vi "Read Dashboard Values.vi"() -> ()   [LabVIEW 2020]
uses:
  <vilib>/Rock Robotics/Network Tables/NT Read Number.vi
  Framework/Robot Global Data.vi
panel:
  out "Auto Drive Time":dbl=3.0 format="%#_13g"
  out "Auto Right Speed":dbl=0.5 format="%#_13g"
  out "Auto Left Speed":dbl=0.5 format="%#_13g"
  out "Auto Shoot Time":dbl=1.0 format="%#_13g"
  out "Auto Shoot Set":dbl=-0.25 format="%#_13g"
  out "Shooter Duration (s)":dbl=3.0 format="%#_13g"
  out "Shooter Setpoint":dbl=0.8 format="%#_13g"
  out "Intake Duration (s)":dbl=3.0 format="%#_13g"
  out "Intake Setpoint":dbl=0.8 format="%#_13g"
  out "Pivot Right Setpoint":dbl=0.4 format="%#_13g"
  out "Pivot Left Setpoint":dbl=0.3 format="%#_13g"
  out "Control Panel Duration (s)":dbl=3.0 format="%#_13g"
  out "Control Panel Setpoint":dbl=0.8 format="%#_13g"
  out "CIimb Duration (s)":dbl=3.0 format="%#_13g"
  out "CIimb Setpoint":dbl=0.8 format="%#_13g"
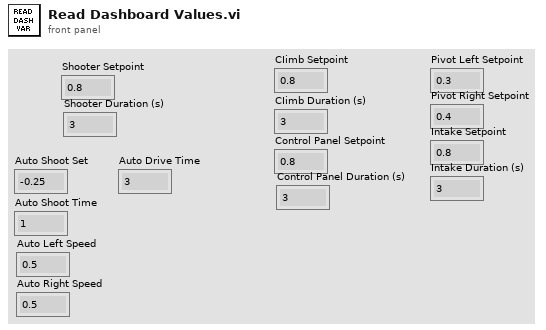
[diagram p1: front panel]
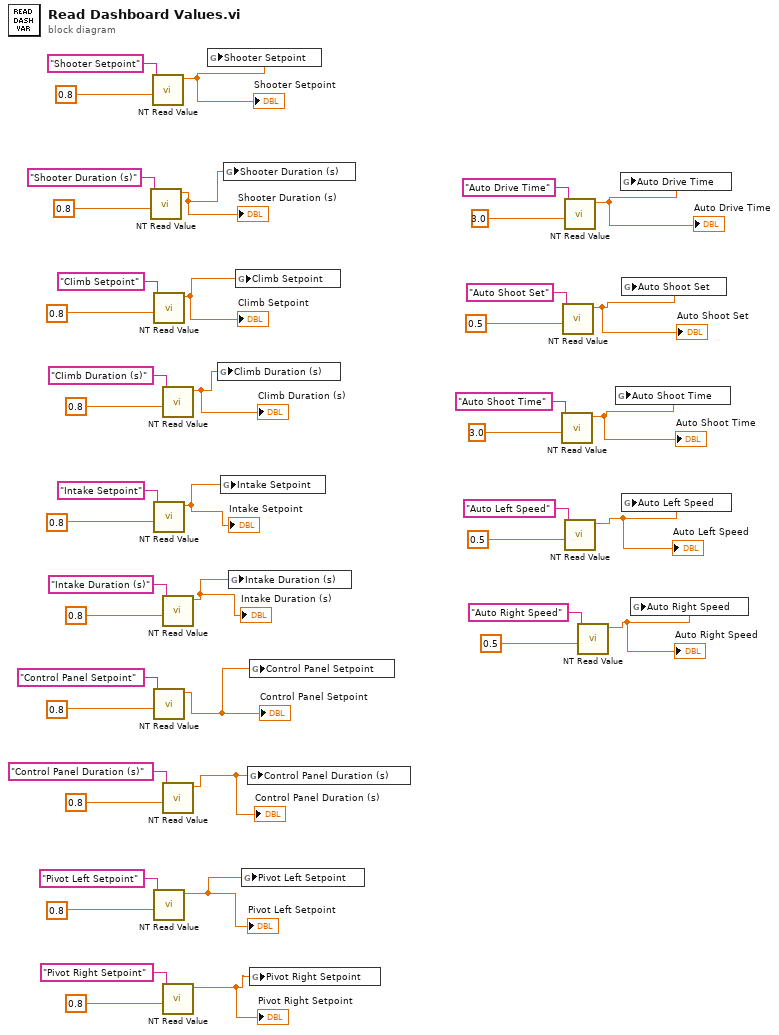
[diagram p0: block diagram]
diagram:
  n1 = call-poly <vilib>:"NT Read Value.vi"("Default Value"=0.8, "Name"="Shooter Duration (s)") -> ("Numeric"=w40:dbl)  [unwired: 8 in, 1 out]
  "Shooter Duration (s)" <- w40
  n2 = call-poly <vilib>:"NT Read Value.vi"("Default Value"=0.8, "Name"="Shooter Setpoint") -> ("Numeric"=w43:dbl)  [unwired: 8 in, 1 out]
  "Shooter Setpoint" <- w43
  n3 = call-poly <vilib>:"NT Read Value.vi"("Default Value"=0.8, "Name"="CIimb Setpoint") -> ("Numeric"=w35:dbl)  [unwired: 8 in, 1 out]
  "CIimb Setpoint" <- w35
  n4 = call-poly <vilib>:"NT Read Value.vi"("Default Value"=0.8, "Name"="Intake Setpoint") -> ("Numeric"=w21:dbl)  [unwired: 8 in, 1 out]
  "Intake Setpoint" <- w21
  n5 = call-poly <vilib>:"NT Read Value.vi"("Default Value"=0.8, "Name"="Control Panel Setpoint") -> ("Numeric"=w18:dbl)  [unwired: 8 in, 1 out]
  "Control Panel Setpoint" <- w18
  n6 = call-poly <vilib>:"NT Read Value.vi"("Default Value"=0.8, "Name"="Pivot Left Setpoint") -> ("Numeric"=w16:dbl)  [unwired: 8 in, 1 out]
  "Pivot Left Setpoint" <- w16
  n7 = call-poly <vilib>:"NT Read Value.vi"("Default Value"=0.8, "Name"="CIimb Duration (s)") -> ("Numeric"=w34:dbl)  [unwired: 8 in, 1 out]
  "CIimb Duration (s)" <- w34
  n8 = call-poly <vilib>:"NT Read Value.vi"("Default Value"=0.8, "Name"="Intake Duration (s)") -> ("Numeric"=w20:dbl)  [unwired: 8 in, 1 out]
  "Intake Duration (s)" <- w20
  n9 = call-poly <vilib>:"NT Read Value.vi"("Default Value"=0.8, "Name"="Control Panel Duration (s)") -> ("Numeric"=w19:dbl)  [unwired: 8 in, 1 out]
  "Control Panel Duration (s)" <- w19
  n10 = call-poly <vilib>:"NT Read Value.vi"("Default Value"=0.8, "Name"="Pivot Right Setpoint") -> ("Numeric"=w17:dbl)  [unwired: 8 in, 1 out]
  "Pivot Right Setpoint" <- w17
  n11 = global write "Robot Global Data.vi" "Shooter Setpoint"(w43) -> ()
  n12 = global write "Robot Global Data.vi" "Climb Duration (s)"(w34) -> ()
  n13 = global write "Robot Global Data.vi" "Intake Setpoint"(w21) -> ()
  n14 = global write "Robot Global Data.vi" "Shooter Duration (s)"(w40) -> ()
  n15 = global write "Robot Global Data.vi" "Intake Duration (s)"(w20) -> ()
  n16 = global write "Robot Global Data.vi" "Climb Setpoint"(w35) -> ()
  n17 = global write "Robot Global Data.vi" "Pivot Left Setpoint"(w16) -> ()
  n18 = global write "Robot Global Data.vi" "Control Panel Duration (s)"(w19) -> ()
  n19 = global write "Robot Global Data.vi" "Control Panel Setpoint"(w18) -> ()
  n20 = global write "Robot Global Data.vi" "Pivot Right Setpoint"(w17) -> ()
  n21 = call-poly <vilib>:"NT Read Value.vi"("Default Value"=3.0, "Name"="Auto Shoot Time") -> ("Numeric"=w3:dbl)  [unwired: 8 in, 1 out]
  "Auto Shoot Time" <- w3
  n22 = call-poly <vilib>:"NT Read Value.vi"("Default Value"=0.5, "Name"="Auto Shoot Set") -> ("Numeric"=w4:dbl)  [unwired: 8 in, 1 out]
  "Auto Shoot Set" <- w4
  n23 = call-poly <vilib>:"NT Read Value.vi"("Default Value"=3.0, "Name"="Auto Drive Time") -> ("Numeric"=w13:dbl)  [unwired: 8 in, 1 out]
  "Auto Drive Time" <- w13
  n24 = call-poly <vilib>:"NT Read Value.vi"("Default Value"=0.5, "Name"="Auto Left Speed") -> ("Numeric"=w2:dbl)  [unwired: 8 in, 1 out]
  "Auto Left Speed" <- w2
  n25 = call-poly <vilib>:"NT Read Value.vi"("Default Value"=0.5, "Name"="Auto Right Speed") -> ("Numeric"=w1:dbl)  [unwired: 8 in, 1 out]
  "Auto Right Speed" <- w1
  n26 = global write "Robot Global Data.vi" "Auto Shoot Time"(w3) -> ()
  n27 = global write "Robot Global Data.vi" "Auto Drive Time"(w13) -> ()
  n28 = global write "Robot Global Data.vi" "Auto Shoot Set"(w4) -> ()
  n29 = global write "Robot Global Data.vi" "Auto Left Speed"(w2) -> ()
  n30 = global write "Robot Global Data.vi" "Auto Right Speed"(w1) -> ()
